vi "水样测试.vi"(10 "数据标记表":string(combo)="N", 11 "水样测试时间":dbl=1.0) -> ()   [LabVIEW 2016, in "斯坦道多参数.lvlib"]
panel:
  out "运行状态":u16(ring) items=["空闲", "水样测试", "标样核查"]
  out "多参数运行日志":string
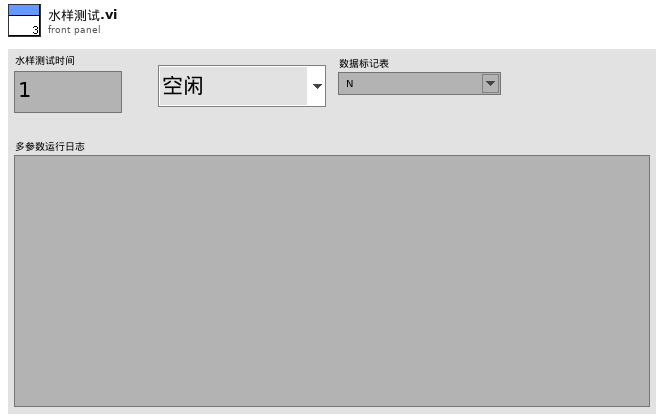
[diagram p1: front panel]
types:
  T1 = cluster{"因子编码":string, "单位":string, "标样参考值":sgl, "水样数据时间":timestamp, "水样实测值":sgl, "水样数据标识":string, "探头温度":sgl}
  T2 = cluster{"温度测量值":sgl, "DO%":sgl, "DOmg/L":sgl, "温度偏移修正值":sgl}
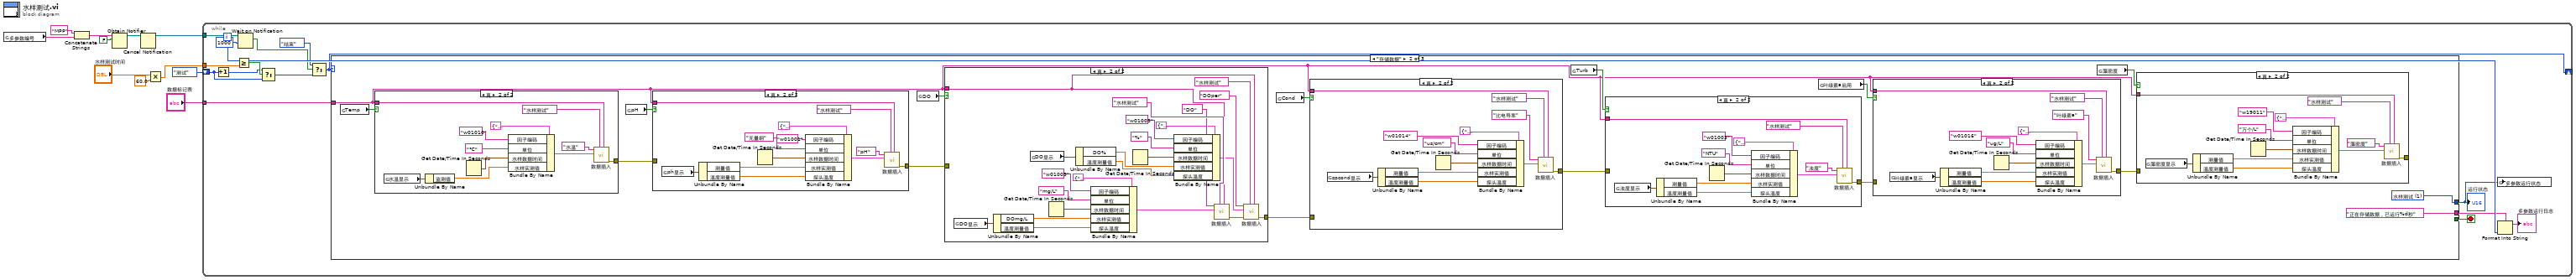
[diagram p0: block diagram]
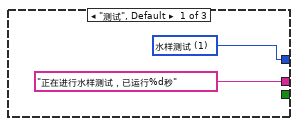
[diagram p2: hidden frame]
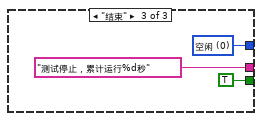
[diagram p10: hidden frame]
diagram:
  n1 = global read "多参数全局变量.vi" "多参数编号"() -> (w1:string)
  n2 = Concatenate Strings("MPP" ("名称（未命名）"), w1) -> (w2:string)
  n3 = Obtain Notifier(name (unnamed)=w2, notification data type=FALSE) -> (notifier out=w5:refnum<notifier>)  [unwired: 2 in, 2 out]
  n4 = Cancel Notification(0:w5) -> (8:w4:refnum<notifier>)  [unwired: 1 in, 2 out]
  n5 = Multiply(x="水样测试时间", y=60.0) -> (x*y=w9:dbl)
  n6 = while {
    tunnel: w9 -> [w27]
    shift-right: [w14] -> _
    shift-left: enum16{"测试", "存储数据", "结束"}."测试" ("枚举") -> [w21]
    tunnel: w4 -> [w19]
    tunnel: "数据标记表" -> [w13]
    i -> [w25]
    stop <- w26 stop-if-true
    n7 = Increment(x=w21) -> (x+1=w20:enum16{"测试", "存储数据", "结束"})
    n8 = Greater Or Equal?(x=w25, y=w27) -> (x >= y?=w22:bool)
    n9 = Wait on Notification(notifier=w19, timeout in ms (-1)=1000 ("超时毫秒(-1)")) -> (notification=w17:bool)  [unwired: 2 in, 3 out]
    n10 = Select(t=w20, s=w22, f=w21) -> (s? t:f=w15:enum16{"测试", "存储数据", "结束"})
    n11 = Select(t=enum16{"测试", "存储数据", "结束"}."结束" ("枚举"), s=w17, f=w15) -> (s? t:f=w14:enum16{"测试", "存储数据", "结束"})
    n12 = case shown="\"存储数据\"" w14 {
      tunnel: [_ _ TRUE] -> w26
      tunnel: ["正在进行水样测试，已运行%d秒" ("格式字符串") "正在存储数据，已运行%d秒" ("格式字符串") "测试停止，累计运行%d秒" ("格式字符串")] -> w24
      tunnel: [w28 w33 w140] -> w12
      tunnel: w13 -> [_ w32 _]
      frame "测试", Default {
        w28 = u16 1 items=["空闲", "水样测试", "标样核查"] ("多参数运行状态")
      }
      frame "存储数据" {
        w33 = u16 1 items=["空闲", "水样测试", "标样核查"] ("多参数运行状态")
        n13 = global read "断电保存变量.vi" "Temp"() -> (w40:bool)
        n14 = case shown="真" w40 {
          tunnel: [_ w132] -> w35
          tunnel: w32 -> [_ w131]
          frame False {
          }
          frame True {
            n15 = global read "多参数全局变量.vi" "水温显示"() -> (w130:cluster{"CH":u16, "监测值":dbl, "温度偏移修正值":sgl})
            n16 = Unbundle By Name(w130) -> ("监测值"=w129:dbl)
            n17 = Get Date/Time In Seconds() -> (seconds since 1Jan1904=w138:timestamp)
            n18 = Bundle By Name(cluster=T1 {"因子编码"="w01003", "单位"="无量纲", "标样参考值"=0.0, "水样数据时间"=timestamp(0 s since 1904-01-01), "水样实测值"=0.0, "水样数据标识"="N", "探头温度"=0.0} ("data in"), "因子编码"="w01010", "单位"="℃", "水样数据时间"=w138, "水样实测值"=w129) -> (w137:T1)
            n19 = call "数据插入.vi"("数据标记表"=w131, "测量模式"="水样测试", "data in"=w137, "table输入"="水温") -> ("error out"=w132:errorcluster)  [unwired: 7 in]
          }
        }
        n20 = global read "断电保存变量.vi" "pH"() -> (w41:bool)
        n21 = case shown="真" w41 {
          tunnel: w35 -> [_ _]
          tunnel: [_ w121] -> w36
          tunnel: w32 -> [_ w120]
          frame False {
          }
          frame True {
            n22 = global read "多参数全局变量.vi" "ph显示"() -> (w119:cluster{"温度测量值":sgl, "测量值":sgl, "温度偏移修正值":sgl})
            n23 = Unbundle By Name(w119) -> ("测量值"=w118:sgl, "温度测量值"=w117:sgl)
            n24 = Get Date/Time In Seconds() -> (seconds since 1Jan1904=w126:timestamp)
            n25 = Bundle By Name(cluster=T1 {"因子编码"="w01003", "单位"="无量纲", "标样参考值"=0.0, "水样数据时间"=timestamp(0 s since 1904-01-01), "水样实测值"=0.0, "水样数据标识"="N", "探头温度"=0.0} ("data in"), "因子编码"="w01001", "单位"="无量纲", "水样数据时间"=w126, "水样实测值"=w118, "探头温度"=w117) -> (w127:T1)
            n26 = call "数据插入.vi"("数据标记表"=w120, "测量模式"="水样测试", "data in"=w127, "table输入"="pH") -> ("error out"=w121:errorcluster)  [unwired: 7 in]
          }
        }
        n27 = global read "断电保存变量.vi" "DO"() -> (w42:bool)
        n28 = case shown="真" w42 {
          tunnel: w36 -> [_ _]
          tunnel: [_ w109] -> w37
          tunnel: w32 -> [_ w107]
          frame False {
          }
          frame True {
            n29 = global read "多参数全局变量.vi" "DO显示"() -> (w98:T2)
            n30 = Unbundle By Name(w98) -> ("DOmg/L"=w97:sgl, "温度测量值"=w96:sgl)
            n31 = global read "多参数全局变量.vi" "DO显示"() -> (w95:T2)
            n32 = Get Date/Time In Seconds() -> (seconds since 1Jan1904=w115:timestamp)
            n33 = Unbundle By Name(w95) -> ("DO%"=w102:sgl, "温度测量值"=w100:sgl)
            n34 = Bundle By Name(cluster=T1 {"因子编码"="w01003", "单位"="无量纲", "标样参考值"=0.0, "水样数据时间"=timestamp(0 s since 1904-01-01), "水样实测值"=0.0, "水样数据标识"="N", "探头温度"=0.0} ("data in"), "因子编码"="w01009", "单位"="mg/L", "水样数据时间"=w115, "水样实测值"=w97, "探头温度"=w96) -> (w114:T1)
            n35 = Get Date/Time In Seconds() -> (seconds since 1Jan1904=w103:timestamp)
            n36 = Bundle By Name(cluster=T1 {"因子编码"="w01003", "单位"="无量纲", "标样参考值"=0.0, "水样数据时间"=timestamp(0 s since 1904-01-01), "水样实测值"=0.0, "水样数据标识"="N", "探头温度"=0.0} ("data in"), "因子编码"="w01009", "单位"="%", "水样数据时间"=w103, "水样实测值"=w102, "探头温度"=w100) -> (w99:T1)
            n37 = call "数据插入.vi"("数据标记表"=w107, "测量模式"="水样测试", "data in"=w114, "table输入"="DO") -> ("error out"=w94:errorcluster)  [unwired: 7 in]
            n38 = call "数据插入.vi"("数据标记表"=w107, "测量模式"="水样测试", "error in (no error)"=w94, "data in"=w99, "table输入"="DOper") -> ("error out"=w109:errorcluster)  [unwired: 6 in]
          }
        }
        n39 = global read "断电保存变量.vi" "Cond"() -> (w43:bool)
        n40 = case shown="真" w43 {
          tunnel: w37 -> [_ _]
          tunnel: [_ w86] -> w38
          tunnel: w32 -> [_ w85]
          frame False {
          }
          frame True {
            n41 = global read "多参数全局变量.vi" "spcond显示"() -> (w84:cluster{"温度测量值":sgl, "测量值":sgl, "温度偏移修正值":sgl})
            n42 = Unbundle By Name(w84) -> ("测量值"=w83:sgl, "温度测量值"=w82:sgl)
            n43 = Get Date/Time In Seconds() -> (seconds since 1Jan1904=w91:timestamp)
            n44 = Bundle By Name(cluster=T1 {"因子编码"="w01003", "单位"="无量纲", "标样参考值"=0.0, "水样数据时间"=timestamp(0 s since 1904-01-01), "水样实测值"=0.0, "水样数据标识"="N", "探头温度"=0.0} ("data in"), "因子编码"="w01014", "单位"="us/cm", "水样数据时间"=w91, "水样实测值"=w83, "探头温度"=w82) -> (w92:T1)
            n45 = call "数据插入.vi"("数据标记表"=w85, "测量模式"="水样测试", "data in"=w92, "table输入"="比电导率") -> ("error out"=w86:errorcluster)  [unwired: 7 in]
          }
        }
        n46 = global read "断电保存变量.vi" "Turb"() -> (w44:bool)
        n47 = case shown="真" w44 {
          tunnel: w38 -> [_ _]
          tunnel: [_ w74] -> w39
          tunnel: w32 -> [_ w73]
          frame False {
          }
          frame True {
            n48 = global read "多参数全局变量.vi" "浊度显示"() -> (w72:cluster{"温度测量值":sgl, "测量值":sgl, "温度偏移修正值":sgl})
            n49 = Unbundle By Name(w72) -> ("测量值"=w71:sgl, "温度测量值"=w70:sgl)
            n50 = Get Date/Time In Seconds() -> (seconds since 1Jan1904=w80:timestamp)
            n51 = Bundle By Name(cluster=T1 {"因子编码"="w01003", "单位"="无量纲", "标样参考值"=0.0, "水样数据时间"=timestamp(0 s since 1904-01-01), "水样实测值"=0.0, "水样数据标识"="N", "探头温度"=0.0} ("data in"), "因子编码"="w01003", "单位"="NTU", "水样数据时间"=w80, "水样实测值"=w71, "探头温度"=w70) -> (w79:T1)
            n52 = call "数据插入.vi"("数据标记表"=w73, "测量模式"="水样测试", "data in"=w79, "table输入"="浊度") -> ("error out"=w74:errorcluster)  [unwired: 7 in]
          }
        }
        n53 = global read "断电保存变量.vi" "叶绿素a启用"() -> (w45:bool)
        n54 = case shown="真" w45 {
          tunnel: w39 -> [_ _]
          tunnel: [_ w60] -> w30
          tunnel: w32 -> [_ w59]
          frame False {
          }
          frame True {
            n55 = global read "多参数全局变量.vi" "叶绿素a显示"() -> (w58:cluster{"温度测量值":sgl, "测量值":sgl, "温度偏移修正值":sgl})
            n56 = Unbundle By Name(w58) -> ("测量值"=w67:sgl, "温度测量值"=w65:sgl)
            n57 = Get Date/Time In Seconds() -> (seconds since 1Jan1904=w68:timestamp)
            n58 = Bundle By Name(cluster=T1 {"因子编码"="w01003", "单位"="无量纲", "标样参考值"=0.0, "水样数据时间"=timestamp(0 s since 1904-01-01), "水样实测值"=0.0, "水样数据标识"="N", "探头温度"=0.0} ("data in"), "因子编码"="w01016", "单位"="ug/L", "水样数据时间"=w68, "水样实测值"=w67, "探头温度"=w65) -> (w63:T1)
            n59 = call "数据插入.vi"("数据标记表"=w59, "测量模式"="水样测试", "data in"=w63, "table输入"="叶绿素a") -> ("error out"=w60:errorcluster)  [unwired: 7 in]
          }
        }
        n60 = global read "断电保存变量.vi" "藻密度"() -> (w31:bool)
        n61 = case shown="真" w31 {
          tunnel: [_ w48] -> _
          tunnel: w32 -> [_ w47]
          tunnel: w30 -> [_ _]
          frame False {
          }
          frame True {
            n62 = global read "多参数全局变量.vi" "藻密度显示"() -> (w46:cluster{"温度测量值":sgl, "测量值":sgl, "温度偏移修正值":sgl})
            n63 = Unbundle By Name(w46) -> ("测量值"=w55:sgl, "温度测量值"=w53:sgl)
            n64 = Get Date/Time In Seconds() -> (seconds since 1Jan1904=w56:timestamp)
            n65 = Bundle By Name(cluster=T1 {"因子编码"="w01003", "单位"="无量纲", "标样参考值"=0.0, "水样数据时间"=timestamp(0 s since 1904-01-01), "水样实测值"=0.0, "水样数据标识"="N", "探头温度"=0.0} ("data in"), "因子编码"="w19011", "单位"="万个/L", "水样数据时间"=w56, "水样实测值"=w55, "探头温度"=w53) -> (w51:T1)
            n66 = call "数据插入.vi"("数据标记表"=w47, "测量模式"="水样测试", "data in"=w51, "table输入"="藻密度") -> ("error out"=w48:errorcluster)  [unwired: 7 in]
          }
        }
      }
      frame "结束" {
        w140 = u16 0 items=["空闲", "水样测试", "标样核查"] ("多参数运行状态")
      }
    }
    "运行状态" <- w12
    n67 = global write "多参数全局变量.vi" "多参数运行状态"(w12) -> ()
    n68 = Format Into String(format string=w24, w25) -> (resulting string=→"多参数运行日志":string)  [unwired: 2 in, 1 out]
  }
